vi "open_or_create_vsd.vi"(8 "error in":errorcluster, 11 "vsd filepath":path) -> (0 "error out":errorcluster, 2 "vsd reference":refnum<k24>, 3 "vsd filepath out":path)   [LabVIEW 2020]
uses:
  NationalInstruments.VeriStand.SystemDefinitionAPI
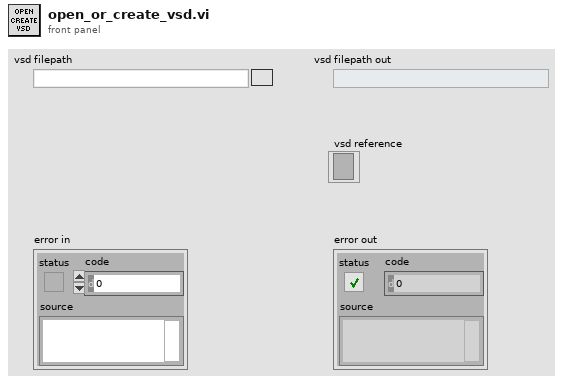
[diagram p1: front panel]
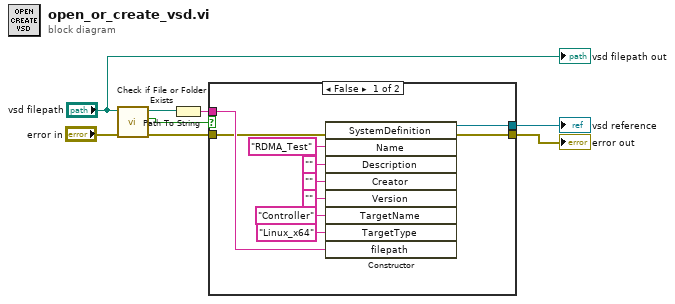
[diagram p0: block diagram]
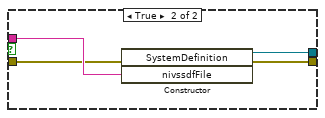
[diagram p2: hidden frame]
diagram:
  n1 = call <vilib>:"Check if File or Folder Exists.vi"("error in (no error)"="error in", "path"="vsd filepath") -> ("error out"=w4:errorcluster, "file or folder exists?"=w8:bool, "dup path"=w7:path)  [unwired: 7 in]
  n2 = Path To String(path=w7) -> (string=w5:string)
  n3 = case shown="False" w8 {
    tunnel: w5 -> [w12 w22]
    tunnel: w4 -> [w11 w21]
    tunnel: [w9 w20] -> w2
    tunnel: [w10 w19] -> w3
    frame False {
      n4 = constructor class="SystemDefinition"(error in=w11, "Name"="RDMA_Test", "Description"="", "Creator"="", "Version"="", "TargetName"="Controller", "TargetType"="Linux_x64", "filepath"=w12) -> (reference out=w10:refnum<k24>, error out=w9:errorcluster)  [unwired: 2 in, 8 out]
    }
    frame True {
      n5 = constructor class="SystemDefinition"(error in=w21, "nivssdfFile"=w22) -> (reference out=w19:refnum<k24>, error out=w20:errorcluster)  [unwired: 2 in, 2 out]
    }
  }
  "vsd reference" <- w3
  "error out" <- w2
  "vsd filepath out" <- "vsd filepath"
